vi "Initialize.vi"(8 "error in (no error)":errorcluster, 10 "Datastrem State":T1, 11 "OXY_SCPI Resource In":refnum<visa-resource-name>) -> (0 "error out":errorcluster, 3 "OXY_SCPI Resource Out":refnum<visa-resource-name>)   [LabVIEW 2020, in "OXYGEN_Datastream.lvlib"]
uses:
  OXYGEN_Datastream.lvlib
  Setup/TypeDefs/States.ctl
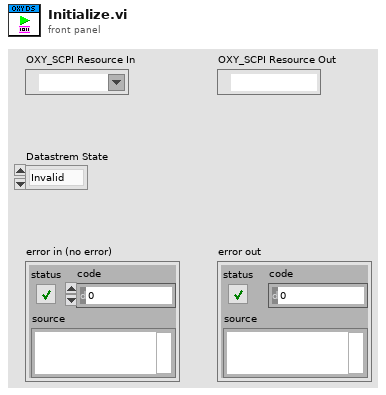
[diagram p1: front panel]
types:
  T1 = typedef "OXYGEN_Datastream.lvlib/States.ctl" = enum16{"Invalid", "Config", "Initialized", "Running", "Error", "Unlicensed"}
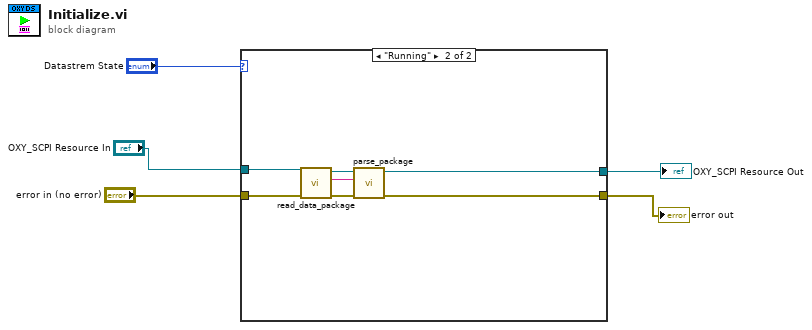
[diagram p0: block diagram]
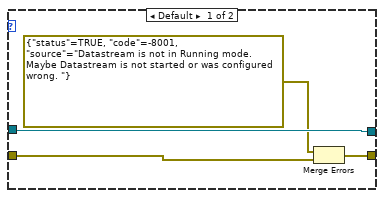
[diagram p2: hidden frame]
diagram:
  n1 = case shown="\"Running\"" "Datastrem State" {
    tunnel: "OXY_SCPI Resource In" -> [w9 w16]
    tunnel: [w9 w13] -> w3
    tunnel: [w8 w12] -> w2
    tunnel: "error in (no error)" -> [w6 w11]
    frame Default {
      n2 = Merge Errors(errorcluster {"status"=TRUE, "code"=-8001, "source"="Datastream is not in Running mode. Maybe Datastream is not started or was configured wrong. "} ("error in"), w6) -> (w8:errorcluster)
    }
    frame "Running" {
      n3 = call "read_data_package.vi"("error in (no error)"=w11, "OXY_SCPI Reseource In"=w16) -> ("error out"=w10:errorcluster, "Package without Header"=w14:string, "OXY_SCPI Reseource Out"=w15:refnum<visa-resource-name>)  [unwired: 6 in, 1 out]
      n4 = call "parse_package.vi"("error in (no error)"=w10, "Raw Package without Header"=w14, "OXY_SCPI Reseource In"=w15) -> ("error out"=w12:errorcluster, "OXY_SCPI Reseource Out"=w13:refnum<visa-resource-name>)  [unwired: 6 in, 1 out]
    }
  }
  "OXY_SCPI Resource Out" <- w3
  "error out" <- w2
